vi "gxml_InsertAttr.vi"(4 "Attribute":string, 5 "Input String":string) -> (2 "Output String":string)   [LabVIEW 2011, in "Third Party VIs.lvlib" / "GXML.lvlib"]
uses:
  GXML.lvlib
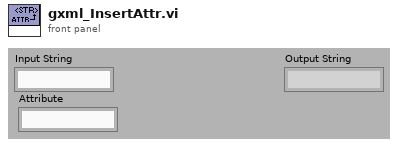
[diagram p1: front panel]
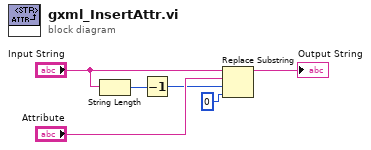
[diagram p0: block diagram]
diagram:
  n1 = String Length(string="Input String") -> (length=w3:i32)
  n2 = Decrement(x=w3) -> (x-1=w2:i32)
  n3 = Replace Substring(2:0 ("length (len. of substring)"), 3:w2, 4:"Attribute", 5:"Input String") -> (1:→"Output String":string)  [unwired: 1 out]
